vi "PhotonPipelineResult_PopulatePacket.vi"(11 "PhotonPipelineResult":T1 {"Targets"."AltCameraToTarget"."TRANSLATION3D"."Z" format="%14.3f"; "Targets"."AltCameraToTarget"."TRANSLATION3D"."Y" format="%14.3f"; "Targets"."AltCameraToTarget"."TRANSLATION3D"."X" format="%14.3f"; "Targets"."BestCameraToTarget"."TRANSLATION3D"."Z" format="%14.3f"; "Targets"."BestCameraToTarget"."TRANSLATION3D"."Y" format="%14.3f"; "Targets"."BestCameraToTarget"."TRANSLATION3D"."X" format="%14.3f"}) -> (3 "Packet_RawData":u8[](array[numeric]))   [LabVIEW 2019, in "PhotonVisionLib.lvlib"]
doc: "Convert a PipelineResult to a Packet array of bytes ready for writing to a Network Table variable.\n\nInputs:\n - PipelineResult -- PipelineResult cluster.\n\nOutputs:\n - Pacet_RawData -- Byte array containing the encoded PipelineResult."
uses:
  PhotonVisionLib.lvlib
  TypeDef/PhotonPipelineResultType.ctl
  TypeDef/PhotonTrackedTargetType.ctl
  TypeDef/TargetCornerType.ctl
  <vilib>/Rock Robotics/WPI/ThirdParty/JAS_Junk/TrajLib/TypeDef/TRANSFORM3D.ctl
  <vilib>/Rock Robotics/WPI/ThirdParty/JAS_Junk/TrajLib/TypeDef/TRANSLATION3D.ctl
  <vilib>/Rock Robotics/WPI/ThirdParty/JAS_Junk/TrajLib/TypeDef/ROTATION3D.ctl
  <vilib>/Rock Robotics/WPI/ThirdParty/JAS_Junk/TrajLib/TypeDef/QUATERNION.ctl
  PhotonTrackedTarget_GetArea.vi
  PhotonTrackedTarget_GetBestCameraToTarget.vi
  PhotonTrackedTarget_GetMinAreaRectCorners.vi
  PhotonTrackedTarget_GetPitch.vi
  PhotonTrackedTarget_GetSkew.vi
  PhotonTrackedTarget_GetYaw.vi
  PhotonTrackedTarget_GetAltCameraToTarget.vi
  Packet_encode_Transform3d.vi
  PhotonTrackedTarget_GetFiducialId.vi
  Packet_encode_Int32.vi
  PhotonTrackedTarget_GetPoseAmbiguity.vi
  PhotonTrackedTarget_GetDetectedCorners.vi
  <vilib>/Rock Robotics/WPI/ThirdParty/JAS_Junk/TrajLib/VI/Transform3d_GetRotation3d.vi
  <vilib>/Rock Robotics/WPI/ThirdParty/JAS_Junk/TrajLib/VI/Transform3d_GetTranslation3d.vi
  <vilib>/Rock Robotics/WPI/ThirdParty/JAS_Junk/TrajLib/VI/Translation3d_ToTranslation2d.vi
  <vilib>/Rock Robotics/WPI/ThirdParty/JAS_Junk/TrajLib/VI/Rotation3d_ToRotation2d.vi
  <vilib>/Rock Robotics/WPI/ThirdParty/JAS_Junk/TrajLib/Transform2d_Create_TransRot.vi
  <vilib>/Rock Robotics/WPI/ThirdParty/JAS_Junk/TrajLib/VI/Transform3d_GetXYZ.vi
  <vilib>/Rock Robotics/WPI/ThirdParty/JAS_Junk/TrajLib/VI/Rotation3d_GetQuaterion.vi
  <vilib>/Rock Robotics/WPI/ThirdParty/JAS_Junk/TrajLib/VI/Quaternion_Get_All.vi
  <vilib>/Rock Robotics/WPI/ThirdParty/JAS_Junk/TrajLib/Translation2d_Create.vi
  <vilib>/Rock Robotics/WPI/ThirdParty/JAS_Junk/TrajLib/Rotation2d_CreateAngle.vi
  <vilib>/Rock Robotics/WPI/ThirdParty/JAS_Junk/TrajLib/VI/Rotation3d_GetXYZ.vi
  <vilib>/Rock Robotics/WPI/ThirdParty/JAS_Junk/TrajLib/VI/Translation3d_GetXYZ.vi
  <vilib>/Rock Robotics/WPI/ThirdParty/JAS_Junk/TrajLib/Trajectory_Library.lvlib
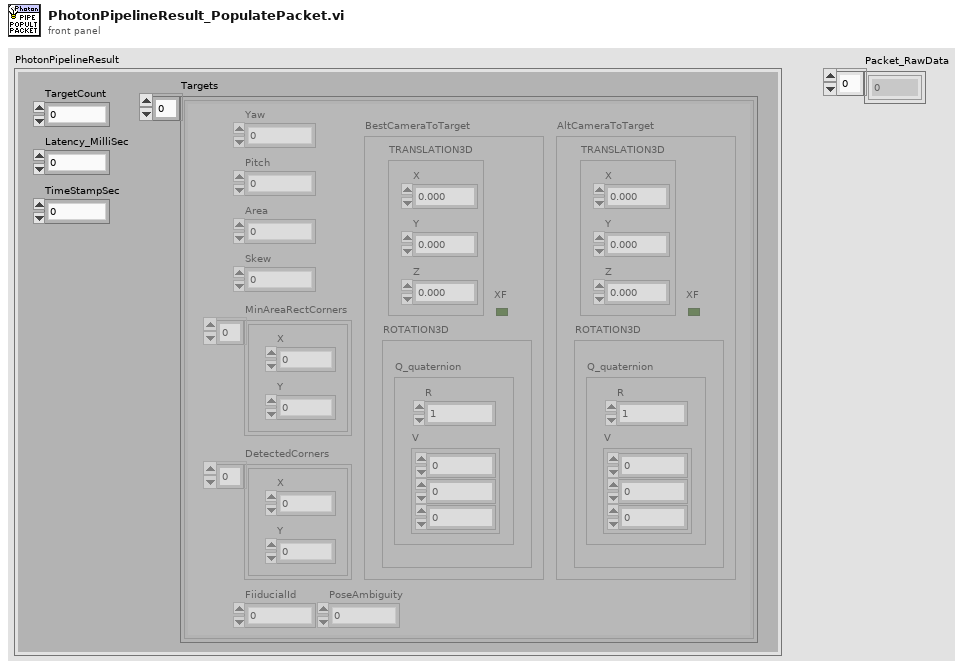
[diagram p1: front panel]
types:
  T1 = typedef "PhotonVisionLib.lvlib/PhotonPipelineResultType.ctl" = cluster{"TargetCount":i32, "Latency_MilliSec":dbl, "Targets":T2[], "TimeStampSec":dbl}
  T2 = typedef "PhotonVisionLib.lvlib/PhotonTrackedTargetType.ctl" = cluster{"Yaw":dbl, "Pitch":dbl, "Area":dbl, "Skew":dbl, "MinAreaRectCorners":T3[], "BestCameraToTarget":T4, "FiiducialId":i32, "AltCameraToTarget":T4, "PoseAmbiguity":dbl, "DetectedCorners":T3[]}
  T3 = typedef "PhotonVisionLib.lvlib/TargetCornerType.ctl" = cluster{"X":dbl, "Y":dbl}
  T4 = typedef "Trajectory_Library.lvlib/TRANSFORM3D.ctl" = cluster{"TRANSLATION3D":T5, "ROTATION3D":T6, "XF":bool}
  T5 = typedef "Trajectory_Library.lvlib/TRANSLATION3D.ctl" = cluster{"X":dbl, "Y":dbl, "Z":dbl}
  T6 = typedef "Trajectory_Library.lvlib/ROTATION3D.ctl" = cluster{"Q_quaternion":T7}
  T7 = typedef "Trajectory_Library.lvlib/QUATERNION.ctl" = cluster{"R":dbl, "V":dbl[]}
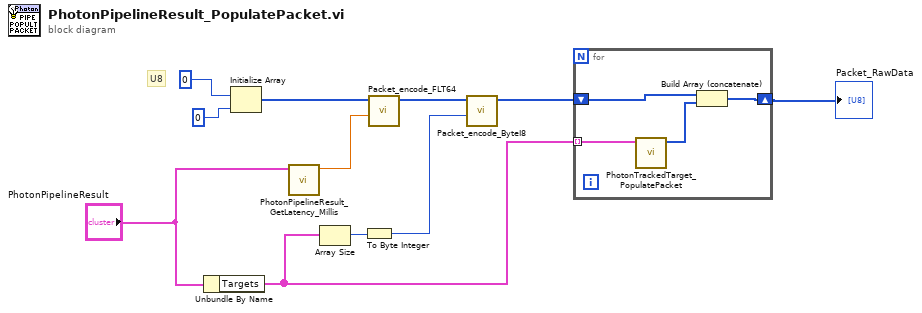
[diagram p0: block diagram]
diagram:
  # "U8"
  n1 = Unbundle By Name("PhotonPipelineResult") -> ("Targets"=w3:T2[])
  n2 = Initialize Array(u8 0 ("element"), 0 ("dimension size")) -> (w7:u8[])
  n3 = call "PhotonPipelineResult_GetLatency_Millis.vi"("PhotonPipelineResult"="PhotonPipelineResult") -> ("Latency_MilliSec"=w6:dbl)  [unwired: 9 in, 1 out]
  n4 = Array Size(array=w3) -> (size(s)=w8:i32)
  n5 = To Byte Integer(number=w8) -> (8bit integer=w4:i8)
  n6 = call "Packet_encode_FLT64.vi"("FLT64_Value"=w6, "RawData In"=w7) -> ("RawData Out"=w5:u8[])  [unwired: 9 in]
  n7 = call "Packet_encode_ByteI8.vi"("Int8_Value"=w4, "RawData In"=w5) -> ("RawData Out"=w2:u8[])  [unwired: 9 in]
  n8 = for {
    tunnel: w3 -> [w15] mode=indexing
    shift-right: [w12] -> w1
    shift-left: w2 -> [w14]
    n9 = call "PhotonTrackedTarget_PopulatePacket.vi"("TrackedTarget"=w15) -> ("RawData Out"=w13:u8[])  [unwired: 10 in]
    n10 = Build Array (concatenate)(w14, w13) -> (w12:u8[])
  }
  "Packet_RawData" <- w1
